vi "Detect Ramp.vi"(3 "Direction":dbl, 5 "Speed":dbl) -> (0 "JoyY":dbl, 1 "Joy X":dbl, 2 "Finished":bool)   [LabVIEW 2014]
uses:
  Begin/Global RefNums.vi
  Begin/Global Variables.vi
  _Dependencies/NavX/navX-MXP IMU.lvlib
panel:
  out "2":cluster{i32, "Pitch":dbl}[](graph)
  out "1":cluster{i32, "Pitch":dbl}[](graph)
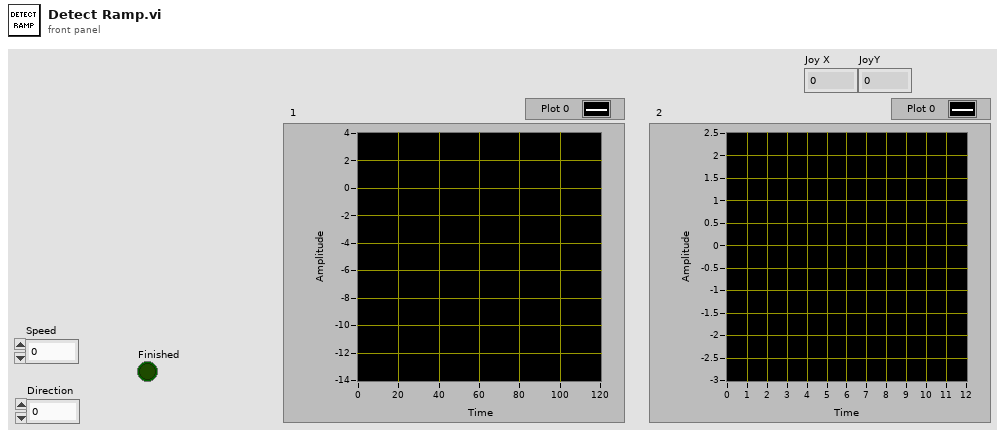
[diagram p1: front panel]
types:
  T1 = typedef "navX-MXP IMU.lvlib/navX Device TypeDef.ctl" = cluster{"navX Interface Protocol":T2, "navX Interface Protocol TypeDefs":cluster{"SPIDevRef":T3, "I2CDevRef":T6}, "navX System Information":cluster{"Board Information":T8, "Status":T9, "Offsets":T13}, "navX Common Information":cluster{"Update Rate (4Hz-60Hz)":T14, "refnum name":string, "error":errorcluster}}
  T2 = typedef "navX-MXP IMU.lvlib/navX Interface Protocol.ctl" = enum16{"SPI", "I2C"}
  T3 = typedef "WPI_SPIDevRef.ctl" = cluster{"DevStatus":errorcluster, "Handle":i32, "Controller":T4, "SPI Bus":T5}
  T4 = typedef "FPGA_TypedefDigitalModule.ctl" = enum16{"Controller 1"}
  T5 = typedef "spi_bus.ctl" = enum16{"SPI On-Board, CS0", "SPI On-Board, CS1", "SPI On-Board, CS2", "SPI On-Board, CS3", "SPI MXP", "Invalid"}
  T6 = typedef "WPI_I2CDevRef.ctl" = cluster{"DevStatus":errorcluster, "Controller":T4, "Device Address":u8, "Handle":i32, "I2C Bus":T7}
  T7 = typedef "i2c_bus.ctl" = enum16{"I2C On-Board", "I2C MXP", "Invalid"}
  T8 = typedef "navX-MXP IMU.lvlib/navX Board Information.ctl" = cluster{"WhoAmI (50 | 0x32)":u8, "Board Revision":u8, "Firmware Major Version":u8, "Firmware Minor Version":u8}
  T9 = typedef "navX-MXP IMU.lvlib/navX Status Data.ctl" = cluster{"Update Rate Hz":u8, "Accelerometer Full-Scale Range":u8, "Gyro Full-Scale Range":u16, "NAVX_OP_STATUS":T10, "NAVX_CAL_STATUS":T11, "NAVX_SELFTEST_STATUS":u8, "NAVX_SENSOR_STATUS":T12}
  T10 = typedef "navX-MXP IMU.lvlib/navX NAVX_OP_STATUS.ctl" = u8
  T11 = typedef "navX-MXP IMU.lvlib/navX NAVX_CAL_STATUS.ctl" = u8
  T12 = typedef "navX-MXP IMU.lvlib/navX NAVX_SENSOR_STATUS.ctl" = cluster{"MOVING":bool, "YAW_STABLE":bool, "MAG_DISTURBANCE":bool, "ALTITUDE_VALID":bool, "SEALEVEL_PRESS_SET":bool, "FUSED_HEADING_VALID":bool}
  T13 = typedef "navX-MXP IMU.lvlib/navX Offsets Data.ctl" = cluster{"Yaw":dbl, "Quat W":dbl, "Quat X":dbl, "Quat Y":dbl, "Quat Z":dbl}
  T14 = typedef "navX-MXP IMU.lvlib/navX Update Rate.ctl" = u8
  T15 = typedef "navX-MXP IMU.lvlib/navX YPRH Data.ctl" = cluster{"Yaw":dbl, "Pitch":dbl, "Roll":dbl, "Heading":dbl}
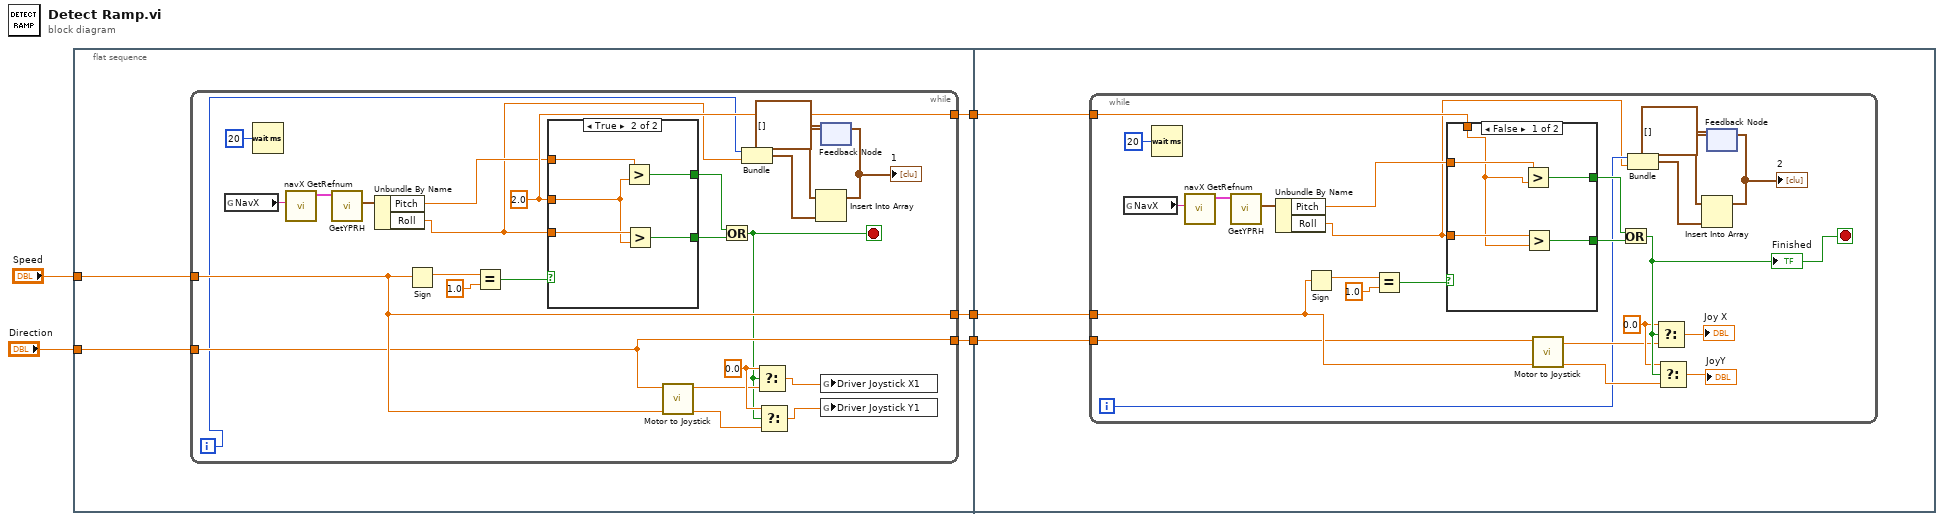
[diagram p0: block diagram]
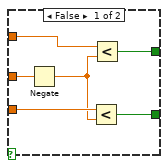
[diagram p2: hidden frame]
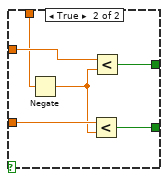
[diagram p3: hidden frame]
diagram:
  n1 = flat-sequence {
    tunnel: [w10] -> w5
    tunnel: "Speed" -> [w9]
    tunnel: "Direction" -> [w8]
    tunnel: [w7] -> w2
    tunnel: [w6] -> w1
    tunnel: w5 -> [w49]
    tunnel: w2 -> [w48]
    tunnel: w1 -> [w47]
    frame #0 {
      n2 = while {
        tunnel: [w26] -> w10
        tunnel: w9 -> [w26]
        tunnel: w8 -> [w25]
        tunnel: [w25] -> w7
        tunnel: [w18] -> w6
        i -> [w17]
        stop <- w20 stop-if-true
        w18 = 2.0 ("y")
        w22 = 0.0 ("t")
        n3 = global read "Global RefNums.vi" "NavX"() -> (w35:string)
        n4 = Wait (ms)(milliseconds to wait=u32 20) -> ()  [unwired: 1 out]
        n5 = call "navX GetRefnum.vi"("refnum name"=w35) -> ("navX Device TypeDef"=w33:T1)  [unwired: 9 in, 1 out]
        n6 = call "GetYPRH.vi"("navX Device TypeDef"=w33) -> ("YPRH"=w34:T15)  [unwired: 8 in, 2 out]
        n7 = Unbundle By Name(w34) -> ("Pitch"=w16:dbl, "Roll"=w11:dbl)
        n8 = Sign(1:w26) -> (0:w29:dbl)
        n9 = Equal?(x=w29, y=1.0) -> (x = y?=w27:bool)
        n10 = case shown="True" w27 {
          tunnel: w16 -> [w41 w46]
          tunnel: w11 -> [w40 w45]
          tunnel: [w39 w44] -> w31
          tunnel: [w38 w43] -> w30
          tunnel: w18 -> [w37 w42]
          frame False {
            n11 = Negate(x=w37) -> (-x=w36:dbl)
            n12 = Less?(x=w40, y=w36) -> (x < y?=w39:bool)
            n13 = Less?(x=w41, y=w36) -> (x < y?=w38:bool)
          }
          frame True {
            n14 = Greater?(x=w46, y=w42) -> (0:w43:bool)
            n15 = Greater?(x=w45, y=w42) -> (0:w44:bool)
          }
        }
        n16 = call "Motor to Joystick.vi"("Drive Motor"=w26, "Rotational Motor"=w25) -> ("Joy Y"=w19:dbl, "Joy X"=w21:dbl)  [unwired: 8 in]
        n17 = Or(x=w30, y=w31) -> (x .or. y?=w20:bool)
        n18 = Bundle(w17, "Roll"=w11) -> (w15:cluster{i32, "Roll":dbl})  [unwired: 1 in]
        n19 = Select(t=w22, s=w20, f=w21) -> (s? t:f=w23:dbl)
        n20 = Select(t=w22, s=w20, f=w19) -> (s? t:f=w24:dbl)
        n21 = feedback #1(cluster{i32, "Pitch":dbl}[] []) -> (w13:cluster{i32, "Pitch":dbl}[])
        n22 = Insert Into Array(array=w13, new element=w15) -> (w14:cluster{i32, "Pitch":dbl}[])  [unwired: 1 in]
        "1" <- w14
        n23 = feedback-in #1(w14) -> ()
        n24 = global write "Global Variables.vi" "Driver Joystick X1"(w23) -> ()
        n25 = global write "Global Variables.vi" "Driver Joystick Y1"(w24) -> ()
      }
    }
    frame #1 {
      n26 = while {
        tunnel: w49 -> [w65]
        tunnel: w48 -> [w64]
        tunnel: w47 -> [w58]
        i -> [w53]
        stop <- w63 stop-if-true
        w62 = 0.0 ("t")
        n27 = global read "Global RefNums.vi" "NavX"() -> (w74:string)
        n28 = Wait (ms)(milliseconds to wait=u32 20) -> ()  [unwired: 1 out]
        n29 = call "navX GetRefnum.vi"("refnum name"=w74) -> ("navX Device TypeDef"=w72:T1)  [unwired: 9 in, 1 out]
        n30 = call "GetYPRH.vi"("navX Device TypeDef"=w72) -> ("YPRH"=w73:T15)  [unwired: 8 in, 2 out]
        n31 = Unbundle By Name(w73) -> ("Pitch"=w59:dbl, "Roll"=w52:dbl)
        n32 = Sign(1:w65) -> (0:w68:dbl)
        n33 = Equal?(x=w68, y=1.0) -> (x = y?=w66:bool)
        n34 = case shown="False" w66 {
          tunnel: w59 -> [w79 w85]
          tunnel: w52 -> [w78 w84]
          tunnel: [w77 w83] -> w70
          tunnel: [w76 w82] -> w69
          tunnel: w58 -> [w75 w80]
          frame False {
            n35 = Greater?(x=w79, y=w75) -> (0:w76:bool)
            n36 = Greater?(x=w78, y=w75) -> (0:w77:bool)
          }
          frame True {
            n37 = Negate(x=w80) -> (-x=w81:dbl)
            n38 = Less?(x=w84, y=w81) -> (x < y?=w83:bool)
            n39 = Less?(x=w85, y=w81) -> (x < y?=w82:bool)
          }
        }
        n40 = call "Motor to Joystick.vi"("Drive Motor"=w65, "Rotational Motor"=w64) -> ("Joy Y"=w61:dbl, "Joy X"=w60:dbl)  [unwired: 8 in]
        n41 = Or(x=w69, y=w70) -> (x .or. y?=w63:bool)
        "Finished" <- w63
        n42 = Bundle(w53, "Roll"=w52) -> (w54:cluster{i32, "Roll":dbl})  [unwired: 1 in]
        n43 = Select(t=w62, s=w63, f=w60) -> (s? t:f=→"Joy X":dbl)
        n44 = Select(t=w62, s=w63, f=w61) -> (s? t:f=→"JoyY":dbl)
        n45 = feedback #2(cluster{i32, "Pitch":dbl}[] []) -> (w56:cluster{i32, "Pitch":dbl}[])
        n46 = Insert Into Array(array=w56, new element=w54) -> (w57:cluster{i32, "Pitch":dbl}[])  [unwired: 1 in]
        "2" <- w57
        n47 = feedback-in #2(w57) -> ()
      }
    }
  }
